vi "Entrada Digital LED.vi"() -> ()   [LabVIEW 2023]
uses:
  <vilib>/Instr/_visa.llb/VISA Configure Serial Port (Instr).vi
panel:
  in  "stop":bool
  in  "ENTRADA COM":refnum<visa-resource-name>
  out "LED":bool
  # "ENTRADA DIGITAL"
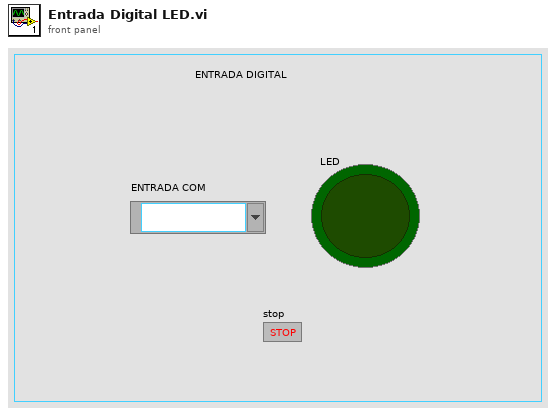
[diagram p1: front panel]
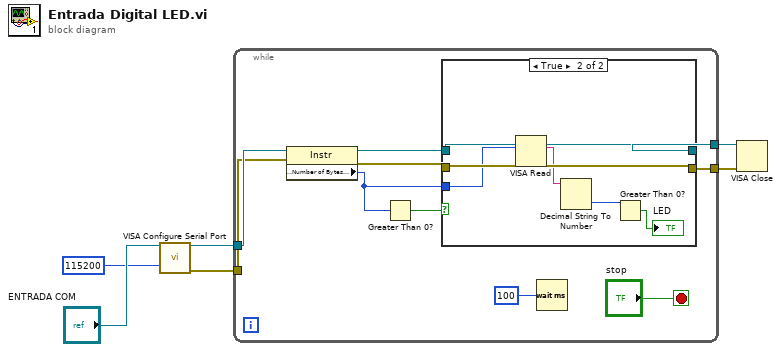
[diagram p0: block diagram]
diagram:
  n1 = call-poly "VISA Configure Serial Port"("VISA resource name"="ENTRADA COM", "baud rate (9600)"=u32 115200) -> ("VISA resource name out"=w5:refnum<visa-resource-name>, "error out"=w4:errorcluster)  [unwired: 12 in]
  n2 = while {
    tunnel: w5 -> [w16]
    tunnel: w4 -> [w15]
    tunnel: [w12] -> w3
    tunnel: [w11] -> w2
    stop <- "stop" stop-if-true
    n3 = property class="Instr"(reference=w16, error in=w15) -> (reference out=w14:refnum<visa-resource-name>, error out=w13:errorcluster, "Serial Settings:Number of Bytes at Serial Port"=w7:u32)
    n4 = Greater Than 0?(x=w7) -> (x > 0?=w8:bool)
    n5 = case shown="True" w8 {
      tunnel: w14 -> [w18 w26]
      tunnel: w13 -> [w17 w25]
      tunnel: [w18 w24] -> w12
      tunnel: [w17 w23] -> w11
      tunnel: w7 -> [_ w22]
      frame False {
      }
      frame True {
        n6 = VISA Read(VISA resource name=w26, byte count=w22, error in (no error)=w25) -> (VISA resource name out=w24:refnum<visa-resource-name>, read buffer=w21:string, error out=w23:errorcluster)  [unwired: 1 out]
        n7 = Decimal String To Number(string=w21) -> (number=w20:i32)  [unwired: 2 in, 1 out]
        n8 = Greater Than 0?(x=w20) -> (x > 0?=→"LED":bool)
      }
    }
    n9 = Wait (ms)(milliseconds to wait=u32 100) -> ()  [unwired: 1 out]
  }
  n10 = VISA Close(VISA resource name=w3, error in (no error)=w2) -> ()  [unwired: 1 out]
